vi "Master2.vi"   [LabVIEW 2016, in "Moving Motor.lvrbt"]
uses:
  Moving Motor.lvrbt
  <vilib>/NXT/Block Support/NXT_InputPort.ctl
  <vilib>/NXT/Hardware/Plugins/Tetrix DC Motor/TetrixDCMotorAddress.ctl
  <vilib>/NXT/Hardware/Plugins/Tetrix 180 deg Servo/Tetrix180ServoAddress.ctl
  <vilib>/NXT/Dual Mode Library/Sensors/EV3_Color_Color.vi
  <vilib>/NXT/NXTIO Xnodes/NXTIONodeSubVIs/TETRIX IO Move Servos.vi
  <vilib>/NXT/NXTIO Xnodes/NXTIONodeSubVIs/TETRIX IO Move DC Motors.vi
  <vilib>/NXT/NXTIO Xnodes/NXTIONodeSubVIs/TETRIX IO Stop DC Motors.vi
  <vilib>/NXT/NXTIO Xnodes/NXTIONodeSubVIs/LEGOStopAllMotors.vi
  <vilib>/NXT/NXTIO Xnodes/AddressXNode/NXTIOAddress.xnode
  <vilib>/NXT/NXTIO Xnodes/NXTIOXNode/NXTIO.xnode
  <vilib>/NXT/Subs/LVHSConnector.ctl
  <vilib>/NXT/LegoClasses/BrickReference/BrickReference.lvclass
types:
  T1 = typedef "NXT_InputPort.ctl" = u32
  T2 = typedef "LVHSConnector.ctl" = refnum<class "BrickReference.lvclass">
  T3 = typedef "Tetrix180ServoAddress.ctl" = i32
  T4 = cluster{"Tetrix180Servo":T3, "Tetrix180Servo":T3}
  T5 = typedef "TetrixDCMotorAddress.ctl" = i32
  T6 = cluster{"TetrixDCMotor":T5, "TetrixDCMotor 2":T5}
  T7 = typedef "ColorSensorColors.ctl" = enum16{"No Color", "Black", "Blue", "Green", "Yellow", "Red", "White", "Brown"}
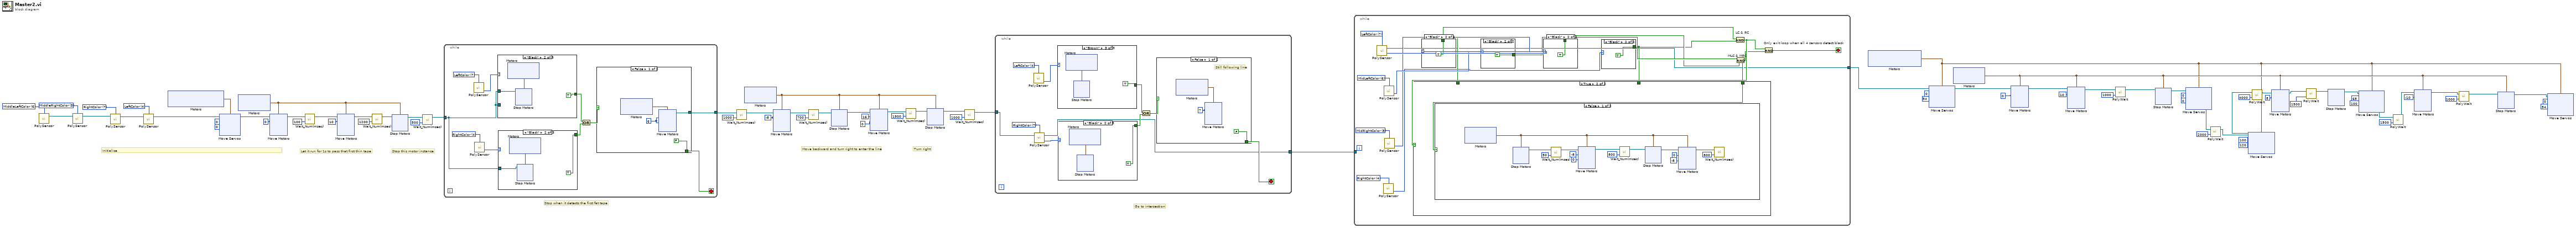
[diagram p0: block diagram]
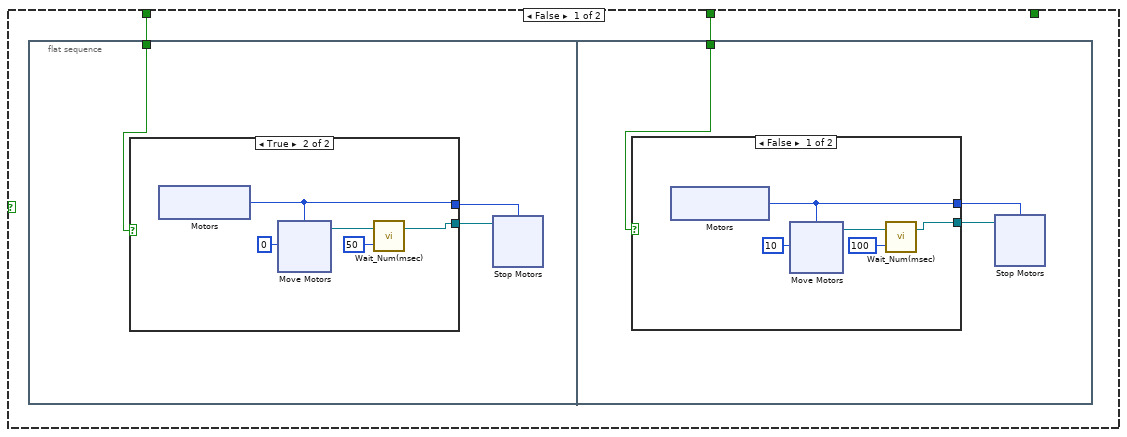
[diagram p2: hidden frame]
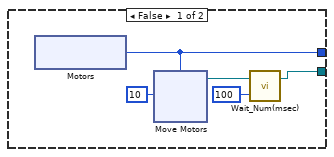
[diagram p3: hidden frame]
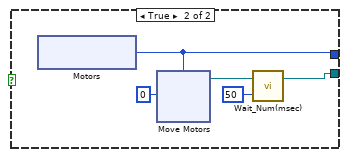
[diagram p4: hidden frame]
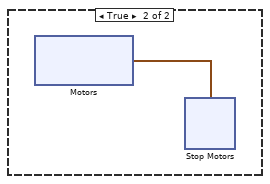
[diagram p5: hidden frame]
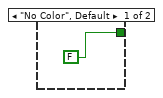
[diagram p6: hidden frame]
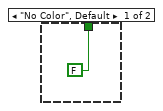
[diagram p7: hidden frame]
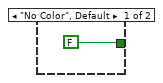
[diagram p8: hidden frame]
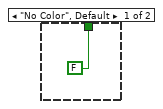
[diagram p9: hidden frame]
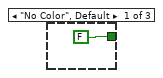
[diagram p10: hidden frame]
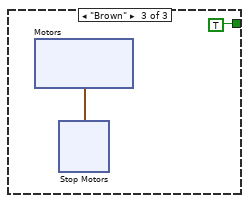
[diagram p11: hidden frame]
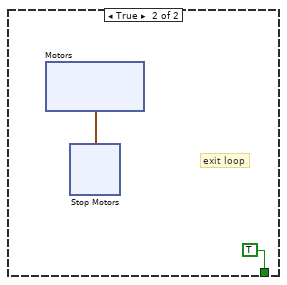
[diagram p12: hidden frame]
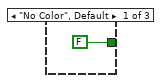
[diagram p13: hidden frame]
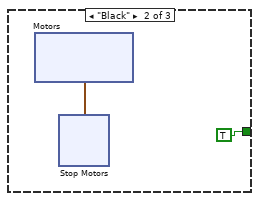
[diagram p14: hidden frame]
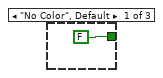
[diagram p15: hidden frame]
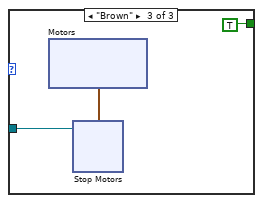
[diagram p16: hidden frame]
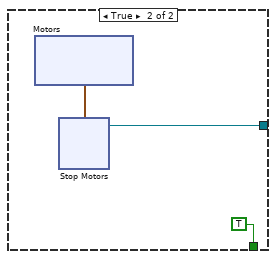
[diagram p17: hidden frame]
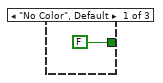
[diagram p18: hidden frame]
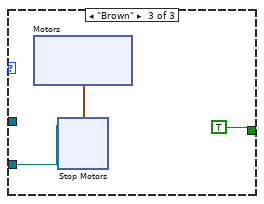
[diagram p19: hidden frame]
diagram:
  w25 = i8 -10 ("Power/Speed 1")
  w27 = i8 8 ("Power/Speed 1")
  w36 = i8 10 ("Power/Speed 1")
  w38 = i8 0 ("Power/Speed 1")
  w43 = T1 6 items=["Port 1"=0, "Port 2"=1, "Port 3"=2, "Port 4"=3, "MiddleLeftColor"=6] ("Port (Port 1)")
  w45 = T1 5 items=["Port 1"=0, "Port 2"=1, "Port 3"=2, "Port 4"=3, "MiddleRightColor"=5] ("Port (Port 1)")
  w52 = T1 7 items=["Port 1"=0, "Port 2"=1, "Port 3"=2, "Port 4"=3, "LeftColor"=4, "RightColor"=7] ("Port (Port 1)")
  w55 = T1 4 items=["Port 1"=0, "Port 2"=1, "Port 3"=2, "Port 4"=3, "LeftColor"=4, "RightColor"=7] ("Port (Port 1)")
  w66 = i8 -8 ("Power/Speed 1")
  w77 = i8 10 ("Power/Speed 1")
  w76 = i8 0 ("Power/Speed 1")
  # "Go to intersection"
  # "Turn right"
  # "Move backward and turn right to enter the line"
  # "Stop this motor instance"
  # "Stop when it detects the first fat tape"
  # "Let it run for 1s to pass that first thin tape"
  # "Initialize"
  n1 = call-poly <vilib>:"PolySensor.vi"("Port (Port 1)"=w43) -> ("NXT/EV3"=w44:T2)  [unwired: 2 in, 1 out]
  n2 = call-poly <vilib>:"PolySensor.vi"("NXT/EV3"=w44, "Port (Port 1)"=w45) -> ("NXT/EV3"=w42:T2)  [unwired: 1 in, 1 out]
  n3 = call-poly <vilib>:"PolySensor.vi"("NXT/EV3"=w42, "Port (Port 1)"=w52) -> ("NXT/EV3"=w53:T2)  [unwired: 1 in, 1 out]
  n4 = call-poly <vilib>:"PolySensor.vi"("NXT/EV3"=w53, "Port (Port 1)"=w55) -> ("NXT/EV3"=w54:T2)  [unwired: 1 in, 1 out]
  n5 = xnode "Motors"() -> ("Motor"=w74:T4)
  n6 = xnode "Move Servos"("Position 2"=u8 0, "Position 1"=u8 0, "Motors"=w74, "NXT/EV3"=w54) -> ("NXT/EV3"=w75:T2)
  n7 = xnode "Motors"() -> ("Motor"=w50:cluster{"TetrixDCMotor":T5, "TetrixDCMotor":T5})
  n8 = xnode "Move Motors"("Power/Speed 2"=w76, "Power/Speed 1"=w76, "Motors"=w50, "NXT/EV3"=w75) -> ("NXT/EV3"=w82:T2)
  n9 = call <vilib>:"Wait_Num(msec).vi"("Time (100 msec)"=u32 100, "NXT/EV3"=w82) -> ("NXT/EV3"=w78:T2)  [unwired: 2 in]
  n10 = xnode "Move Motors"("Power/Speed 2"=w77, "Power/Speed 1"=w77, "Motors"=w50, "NXT/EV3"=w78) -> ("NXT/EV3"=w80:T2)
  n11 = call <vilib>:"Wait_Num(msec).vi"("Time (100 msec)"=u32 1200, "NXT/EV3"=w80) -> ("NXT/EV3"=w51:T2)  [unwired: 2 in]
  n12 = xnode "Stop Motors"("Motors"=w50, "NXT/EV3"=w51) -> ("NXT/EV3"=w48:T2)
  n13 = call <vilib>:"Wait_Num(msec).vi"("Time (100 msec)"=u32 500, "NXT/EV3"=w48) -> ("NXT/EV3"=w47:T2)  [unwired: 2 in]
  n14 = while {
    tunnel: [w86] -> w68
    tunnel: w47 -> [w83]
    stop <- w87 stop-if-true
    w90 = T1 4 items=["Port 1", "Port 2", "Port 3", "Port 4", "RightColor"] ("Port (Port 1)")
    w92 = T1 7 items=["Port 1"=0, "Port 2"=1, "Port 3"=2, "Port 4"=3, "LeftColor"=7] ("Port (Port 1)")
    n15 = call-poly <vilib>:"PolySensor.vi"("Port (Port 1)"=w92) -> ("Detected Color"=w91:T7)  [unwired: 2 in, 1 out]
    n16 = call-poly <vilib>:"PolySensor.vi"("Port (Port 1)"=w90) -> ("Detected Color"=w89:T7)  [unwired: 2 in, 1 out]
    n17 = case shown="\"Black\"" w91 {
      tunnel: [FALSE TRUE TRUE] -> w85
      tunnel: w83 -> [_ w135 _]
      tunnel: w83 -> [_ _ w144]
      frame "No Color", Default {
      }
      frame "Black" {
        n18 = xnode "Motors"() -> ("Motor"=w137:cluster{"TetrixDCMotor":T5, "TetrixDCMotor":T5})
        n19 = xnode "Stop Motors"("Motors"=w137, "NXT/EV3"=w135) -> ()  [unwired: 1 out]
      }
      frame "Brown" {
        n20 = xnode "Motors"() -> ("Motor"=w145:cluster{"TetrixDCMotor":T5, "TetrixDCMotor":T5})
        n21 = xnode "Stop Motors"("Motors"=w145, "NXT/EV3"=w144) -> ()  [unwired: 1 out]
      }
    }
    n22 = case shown="\"Black\"" w89 {
      tunnel: [FALSE TRUE TRUE] -> w84
      tunnel: w83 -> [_ w94 w103]
      frame "No Color", Default {
      }
      frame "Black" {
        n23 = xnode "Motors"() -> ("Motor"=w95:cluster{"TetrixDCMotor":T5, "TetrixDCMotor":T5})
        n24 = xnode "Stop Motors"("Motors"=w95, "NXT/EV3"=w94) -> ()  [unwired: 1 out]
      }
      frame "Brown" {
        n25 = xnode "Motors"() -> ("Motor"=w104:cluster{"TetrixDCMotor":T5, "TetrixDCMotor":T5})
        n26 = xnode "Stop Motors"("Motors"=w104, "NXT/EV3"=w103) -> ()  [unwired: 1 out]
      }
    }
    n27 = Or(x=w85, y=w84) -> (x .or. y?=w88:bool)
    n28 = case shown="False" w88 {
      tunnel: [FALSE TRUE] -> w87
      tunnel: [w112 w125] -> w86
      frame False {
        w115 = i8 6 ("Power/Speed 1")
        n29 = xnode "Motors"() -> ("Motor"=w114:cluster{"TetrixDCMotor":T5, "TetrixDCMotor":T5})
        n30 = xnode "Move Motors"("Power/Speed 2"=w115, "Power/Speed 1"=w115, "Motors"=w114) -> ("NXT/EV3"=w112:T2)  [unwired: 1 in]
      }
      frame True {
        n31 = xnode "Motors"() -> ("Motor"=w126:cluster{"TetrixDCMotor":T5, "TetrixDCMotor":T5})
        n32 = xnode "Stop Motors"("Motors"=w126) -> ("NXT/EV3"=w125:T2)  [unwired: 1 in]
      }
    }
  }
  n33 = call <vilib>:"Wait_Num(msec).vi"("Time (100 msec)"=u32 1000, "NXT/EV3"=w68) -> ("NXT/EV3"=w67:T2)  [unwired: 2 in]
  n34 = xnode "Motors"() -> ("Motor"=w59:cluster{"TetrixDCMotor":T5, "TetrixDCMotor":T5})
  n35 = xnode "Move Motors"("Power/Speed 2"=w66, "Power/Speed 1"=w66, "Motors"=w59, "NXT/EV3"=w67) -> ("NXT/EV3"=w64:T2)
  n36 = call <vilib>:"Wait_Num(msec).vi"("Time (100 msec)"=u32 700, "NXT/EV3"=w64) -> ("NXT/EV3"=w60:T2)  [unwired: 2 in]
  n37 = xnode "Stop Motors"("Motors"=w59, "NXT/EV3"=w60) -> ("NXT/EV3"=w58:T2)
  n38 = xnode "Move Motors"("Power/Speed 2"=i8 0, "Power/Speed 1"=i8 16, "Motors"=w59, "NXT/EV3"=w58) -> ("NXT/EV3"=w61:T2)
  n39 = call <vilib>:"Wait_Num(msec).vi"("Time (100 msec)"=u32 1900, "NXT/EV3"=w61) -> ("NXT/EV3"=w70:T2)  [unwired: 2 in]
  n40 = xnode "Stop Motors"("Motors"=w59, "NXT/EV3"=w70) -> ("NXT/EV3"=w56:T2)
  n41 = call <vilib>:"Wait_Num(msec).vi"("Time (100 msec)"=u32 1000, "NXT/EV3"=w56) -> ("NXT/EV3"=w46:T2)  [unwired: 2 in]
  n42 = while {
    tunnel: [w154] -> w41
    tunnel: w46 -> [w153]
    stop <- w157 stop-if-true
    w160 = T1 7 items=["Port 1"=0, "Port 2"=1, "Port 3"=2, "Port 4"=3, "LeftColor"=4, "RightColor"=7] ("Port (Port 1)")
    w162 = T1 4 items=["Port 1"=0, "Port 2"=1, "Port 3"=2, "Port 4"=3, "LeftColor"=4, "RightColor"=7] ("Port (Port 1)")
    n43 = call-poly <vilib>:"PolySensor.vi"("Port (Port 1)"=w162) -> ("Detected Color"=w161:T7)  [unwired: 2 in, 1 out]
    n44 = call-poly <vilib>:"PolySensor.vi"("NXT/EV3"=w153, "Port (Port 1)"=w160) -> ("Detected Color"=w159:T7, "NXT/EV3"=w154:T2)  [unwired: 1 in]
    n45 = case shown="\"Brown\"" w161 {
      tunnel: [FALSE TRUE TRUE] -> w156
      frame "No Color", Default {
      }
      frame "Black" {
        n46 = xnode "Motors"() -> ("Motor"=w202:cluster{"TetrixDCMotor":T5, "TetrixDCMotor":T5})
        n47 = xnode "Stop Motors"("Motors"=w202) -> ()  [unwired: 1 in, 1 out]
      }
      frame "Brown" {
        n48 = xnode "Motors"() -> ("Motor"=w209:cluster{"TetrixDCMotor":T5, "TetrixDCMotor":T5})
        n49 = xnode "Stop Motors"("Motors"=w209) -> ()  [unwired: 1 in, 1 out]
      }
    }
    n50 = case shown="\"Black\"" w159 {
      tunnel: [FALSE TRUE TRUE] -> w155
      frame "No Color", Default {
      }
      frame "Black" {
        n51 = xnode "Motors"() -> ("Motor"=w164:cluster{"TetrixDCMotor":T5, "TetrixDCMotor":T5})
        n52 = xnode "Stop Motors"("Motors"=w164) -> ()  [unwired: 1 in, 1 out]
      }
      frame "Brown" {
        n53 = xnode "Motors"() -> ("Motor"=w172:cluster{"TetrixDCMotor":T5, "TetrixDCMotor":T5})
        n54 = xnode "Stop Motors"("Motors"=w172) -> ()  [unwired: 1 in, 1 out]
      }
    }
    n55 = Or(x=w156, y=w155) -> (x .or. y?=w158:bool)
    n56 = case shown="False" w158 {
      tunnel: [FALSE TRUE] -> w157
      frame False {
        w181 = i8 7 ("Power/Speed 1")
        # "Still following line"
        n57 = xnode "Motors"() -> ("Motor"=w180:cluster{"TetrixDCMotor":T5, "TetrixDCMotor":T5})
        n58 = xnode "Move Motors"("Power/Speed 2"=w181, "Power/Speed 1"=w181, "Motors"=w180) -> ()  [unwired: 1 in, 1 out]
      }
      frame True {
        # "exit loop"
        n59 = xnode "Motors"() -> ("Motor"=w192:cluster{"TetrixDCMotor":T5, "TetrixDCMotor":T5})
        n60 = xnode "Stop Motors"("Motors"=w192) -> ()  [unwired: 1 in, 1 out]
      }
    }
  }
  n61 = while {
    tunnel: w41 -> [_]
    tunnel: [w217] -> w1
    stop <- w218 stop-if-true
    w229 = T1 5 items=["Port 1"=0, "Port 2"=1, "Port 3"=2, "Port 4"=3, "MidRightColor"=5] ("Port (Port 1)")
    w230 = T1 6 items=["Port 1"=0, "Port 2"=1, "Port 3"=2, "Port 4"=3, "MidLeftColor"=6] ("Port (Port 1)")
    w231 = T1 4 items=["Port 1", "Port 2", "Port 3", "Port 4", "RightColor"] ("Port (Port 1)")
    w232 = T1 7 items=["Port 1"=0, "Port 2"=1, "Port 3"=2, "Port 4"=3, "LeftColor"=7] ("Port (Port 1)")
    n62 = call-poly <vilib>:"PolySensor.vi"("Port (Port 1)"=w232) -> ("Detected Color"=w228:T7, "NXT/EV3"=w217:T2)  [unwired: 2 in]
    n63 = call-poly <vilib>:"PolySensor.vi"("Port (Port 1)"=w231) -> ("Detected Color"=w225:T7)  [unwired: 2 in, 1 out]
    n64 = call-poly <vilib>:"PolySensor.vi"("Port (Port 1)"=w230) -> ("Detected Color"=w227:T7)  [unwired: 2 in, 1 out]
    n65 = call-poly <vilib>:"PolySensor.vi"("Port (Port 1)"=w229) -> ("Detected Color"=w226:T7)  [unwired: 2 in, 1 out]
    n66 = case shown="\"Black\"" w228 {
      tunnel: [FALSE TRUE] -> w221
      frame "No Color", Default {
      }
      frame "Black" {
      }
    }
    n67 = case shown="\"Black\"" w227 {
      tunnel: [FALSE TRUE] -> w224
      frame "No Color", Default {
      }
      frame "Black" {
      }
    }
    n68 = case shown="\"Black\"" w226 {
      tunnel: [FALSE TRUE] -> w223
      frame "No Color", Default {
      }
      frame "Black" {
      }
    }
    n69 = case shown="\"Black\"" w225 {
      tunnel: [FALSE TRUE] -> w220
      frame "No Color", Default {
      }
      frame "Black" {
      }
    }
    n70 = And "LC & RC"(x=w221, y=w220) -> (x .and. y?=w222:bool)
    n71 = And "MLC & MRC"(x=w224, y=w223) -> (x .and. y?=w219:bool)
    n72 = case shown="True" w222 {
      tunnel: w221 -> [w234 _]
      tunnel: w220 -> [w233 _]
      tunnel: w219 -> [_ w303]
      frame False {
        n73 = flat-sequence {
          tunnel: w234 -> [w235]
          tunnel: w233 -> [w269]
          frame #0 {
            n74 = case shown="True" w235 {
              tunnel: [w244 w256] -> w237
              tunnel: [w243 w257] -> w236
              frame False {
                n75 = xnode "Motors"() -> ("Motor"=w243:T5)
                n76 = xnode "Move Motors"("Power/Speed 1"=i8 10, "Motors"=w243) -> ("NXT/EV3"=w246:T2)  [unwired: 1 in]
                n77 = call <vilib>:"Wait_Num(msec).vi"("Time (100 msec)"=u32 100, "NXT/EV3"=w246) -> ("NXT/EV3"=w244:T2)  [unwired: 2 in]
              }
              frame True {
                n78 = xnode "Motors"() -> ("Motor"=w257:T5)
                n79 = xnode "Move Motors"("Power/Speed 1"=i8 0, "Motors"=w257) -> ("NXT/EV3"=w259:T2)  [unwired: 1 in]
                n80 = call <vilib>:"Wait_Num(msec).vi"("Time (100 msec)"=u32 50, "NXT/EV3"=w259) -> ("NXT/EV3"=w256:T2)  [unwired: 2 in]
              }
            }
            n81 = xnode "Stop Motors"("Motors"=w236, "NXT/EV3"=w237) -> ()  [unwired: 1 out]
          }
          frame #1 {
            n82 = case shown="False" w269 {
              tunnel: [w278 w290] -> w271
              tunnel: [w277 w291] -> w270
              frame False {
                n83 = xnode "Motors"() -> ("Motor"=w277:T5)
                n84 = xnode "Move Motors"("Power/Speed 1"=i8 10, "Motors"=w277) -> ("NXT/EV3"=w280:T2)  [unwired: 1 in]
                n85 = call <vilib>:"Wait_Num(msec).vi"("Time (100 msec)"=u32 100, "NXT/EV3"=w280) -> ("NXT/EV3"=w278:T2)  [unwired: 2 in]
              }
              frame True {
                n86 = xnode "Motors"() -> ("Motor"=w291:T5)
                n87 = xnode "Move Motors"("Power/Speed 1"=i8 0, "Motors"=w291) -> ("NXT/EV3"=w293:T2)  [unwired: 1 in]
                n88 = call <vilib>:"Wait_Num(msec).vi"("Time (100 msec)"=u32 50, "NXT/EV3"=w293) -> ("NXT/EV3"=w290:T2)  [unwired: 2 in]
              }
            }
            n89 = xnode "Stop Motors"("Motors"=w270, "NXT/EV3"=w271) -> ()  [unwired: 1 out]
          }
        }
      }
      frame True {
        n90 = case shown="False" w303 {
          frame False {
            n91 = xnode "Motors"() -> ("Motor"=w309:cluster{"TetrixDCMotor":T5, "TetrixDCMotor":T5})
            n92 = xnode "Stop Motors"("Motors"=w309) -> ("NXT/EV3"=w315:T2)  [unwired: 1 in]
            n93 = call <vilib>:"Wait_Num(msec).vi"("Time (100 msec)"=u32 50, "NXT/EV3"=w315) -> ("NXT/EV3"=w310:T2)  [unwired: 2 in]
            n94 = xnode "Move Motors"("Power/Speed 2"=i8 0, "Power/Speed 1"=i8 -8, "Motors"=w309, "NXT/EV3"=w310) -> ("NXT/EV3"=w312:T2)
            n95 = call <vilib>:"Wait_Num(msec).vi"("Time (100 msec)"=u32 800, "NXT/EV3"=w312) -> ("NXT/EV3"=w316:T2)  [unwired: 2 in]
            n96 = xnode "Stop Motors"("Motors"=w309, "NXT/EV3"=w316) -> ("NXT/EV3"=w306:T2)
            n97 = xnode "Move Motors"("Power/Speed 2"=i8 -8, "Power/Speed 1"=i8 0, "Motors"=w309, "NXT/EV3"=w306) -> ("NXT/EV3"=w304:T2)
            n98 = call <vilib>:"Wait_Num(msec).vi"("Time (100 msec)"=u32 800, "NXT/EV3"=w304) -> ()  [unwired: 2 in, 1 out]
          }
          frame True {
            n99 = xnode "Motors"() -> ("Motor"=w345:cluster{"TetrixDCMotor":T5, "TetrixDCMotor":T5})
            n100 = xnode "Stop Motors"("Motors"=w345) -> ()  [unwired: 1 in, 1 out]
          }
        }
      }
    }
    n101 = And "Only exit loop when all 4 sensors detect black"(x=w222, y=w219) -> (x .and. y?=w218:bool)
  }
  n102 = xnode "Motors"() -> ("Motor"=w8:T4)
  n103 = xnode "Move Servos"("Position 2"=u8 54, "Position 1"=u8 0, "Motors"=w8, "NXT/EV3"=w1) -> ("NXT/EV3"=w37:T2)
  n104 = xnode "Motors"() -> ("Motor"=w19:cluster{"TetrixDCMotor":T5, "TetrixDCMotor":T5})
  n105 = xnode "Move Motors"("Power/Speed 2"=w38, "Power/Speed 1"=w38, "Motors"=w19, "NXT/EV3"=w37) -> ("NXT/EV3"=w33:T2)
  n106 = xnode "Move Motors"("Power/Speed 2"=w36, "Power/Speed 1"=w36, "Motors"=w19, "NXT/EV3"=w33) -> ("NXT/EV3"=w34:T2)
  n107 = call-poly <vilib>:"PolyWait.vi"("Time (100 msec)"=u32 1000, "NXT/EV3"=w34) -> ("NXT/EV3"=w32:T2)  [unwired: 2 in]
  n108 = xnode "Stop Motors"("Motors"=w19, "NXT/EV3"=w32) -> ("NXT/EV3"=w9:T2)
  n109 = xnode "Move Servos"("Position 2"=u8 0, "Position 1"=u8 0, "Motors"=w8, "NXT/EV3"=w9) -> ("NXT/EV3"=w4:T2)
  n110 = call-poly <vilib>:"PolyWait.vi"("Time (100 msec)"=u32 2000, "NXT/EV3"=w4) -> ("NXT/EV3"=w3:T2)  [unwired: 2 in]
  n111 = xnode "Move Servos"("Position 2"=u8 120, "Position 1"=u8 100, "Motors"=w8, "NXT/EV3"=w3) -> ("NXT/EV3"=w2:T2)
  n112 = call-poly <vilib>:"PolyWait.vi"("Time (100 msec)"=u32 4000, "NXT/EV3"=w2) -> ("NXT/EV3"=w13:T2)  [unwired: 2 in]
  n113 = xnode "Move Motors"("Power/Speed 2"=w27, "Power/Speed 1"=w27, "Motors"=w19, "NXT/EV3"=w13) -> ("NXT/EV3"=w24:T2)
  n114 = call-poly <vilib>:"PolyWait.vi"("Time (100 msec)"=u32 1500, "NXT/EV3"=w24) -> ("NXT/EV3"=w23:T2)  [unwired: 2 in]
  n115 = xnode "Stop Motors"("NXT/EV3"=w23) -> ("NXT/EV3"=w22:T2)  [unwired: 1 in]
  n116 = xnode "Move Servos"("Position 2"=u8 100, "Position 1"=u8 65, "Motors"=w8, "NXT/EV3"=w22) -> ("NXT/EV3"=w11:T2)
  n117 = call-poly <vilib>:"PolyWait.vi"("Time (100 msec)"=u32 1500, "NXT/EV3"=w11) -> ("NXT/EV3"=w10:T2)  [unwired: 2 in]
  n118 = xnode "Move Motors"("Power/Speed 2"=w25, "Power/Speed 1"=w25, "Motors"=w19, "NXT/EV3"=w10) -> ("NXT/EV3"=w21:T2)
  n119 = call-poly <vilib>:"PolyWait.vi"("Time (100 msec)"=u32 1000, "NXT/EV3"=w21) -> ("NXT/EV3"=w18:T2)  [unwired: 2 in]
  n120 = xnode "Stop Motors"("Motors"=w19, "NXT/EV3"=w18) -> ("NXT/EV3"=w17:T2)
  n121 = xnode "Move Servos"("Position 2"=u8 54, "Position 1"=u8 0, "Motors"=w8, "NXT/EV3"=w17) -> ()  [unwired: 1 out]
